vi "RT Main.vi"   [LabVIEW 2018]
doc: "Main real-time VI running on cRIO"
uses:
  Support/Message Queue/Message.ctl
  Controls/Control Mode.ctl
  Controls/Parameters.ctl
  Controls/Config.ctl
  Controls/Settings.ctl
  Controls/Timeouts.ctl
  Controls/ConfigCalibration.ctl
  Controls/ValveState.ctl
  Controls/Valve List.ctl
  Controls/ValveUpdate.ctl
  Controls/IT State.ctl
  Controls/OT State.ctl
  Controls/DL State.ctl
  Controls/BR State.ctl
  Controls/TWT State.ctl
  Controls/DLT State.ctl
  Controls/Clean State.ctl
  Controls/Actions.ctl
  Globals/Global - Configuration Options.vi
  Globals/Global - RT Stream Connections.vi
  support/Message Queue/Message Queue.lvlib
  <vilib>/nisyscfg/nisyscfg.lvlib
types:
  T1 = typedef "Message Queue.lvlib/Message.ctl" = enum16{"Initialize", "Initialize UI Refs", "Disable Controls", "Enable UI Controls", "Connect RT", "Get Control Mode from RT", "Send Control Mode to UI", "Update Control Mode", "Get Config from RT", "Send Config to UI", "Update Parameters", "Change Parameters", "Calibrate Config", "Update Calibration", "Change Valve State", "Get Valve Status from RT", "Send Valve Status to UI", "Update Valve Status", "Inital UI Values", "Disconnect RT", "Close Connection", "Disconnect UI", "Run Mode", "Stop ALL", "Change Control Mode", "Skid Manual", "Computer Manual", "Step Automated", "Fully Automated", "Reset", "Critical Error", "Log-Only Error", "Non-Critical Error", "RT Error", "Update System Status", "Update DI Status", "Clear System Status", "Update Warning", "Clear Warning", "Upate Timeout", "Update Reset Status", "Waiting", "Verify Password", "Manual Cleaning Process", "Update Manual Cleaning Process", "Exit", "---Copy This Frame---"}
  T2 = typedef "Control Mode.ctl" = enum16{"Skid Manual", "Computer Manual", "Step Automated", "Fully Automated"}
  T3 = typedef "Parameters.ctl" = cluster{"PDP (IN)":T4, "SETTINGS":T5, "TIMEOUTS (SEC)":T6}
  T4 = typedef "Config.ctl" = cluster{"TWTT OP":dbl, "TWTT PDP":dbl, "DLT OP":dbl, "DLT PDP 01":dbl, "DLT PDP 02":dbl, "BR OP":dbl, "BR TWT ALIGN":dbl, "BR DL ALIGN":dbl}
  T5 = typedef "Settings.ctl" = cluster{"HPL Low (PSI)":dbl, "HPL High (PSI)":dbl, "HPH Low (PSI)":dbl, "HPH High (PSI)":dbl, "AP Low (PSI)":dbl, "AP High (PSI)":dbl, "DL Clean (SEC)":dbl, "Reset (MIN)":dbl}
  T6 = typedef "Timeouts.ctl" = cluster{"TWTT Drive":dbl, "DL Drive":dbl, "DL Rotate":dbl, "BR Drive":dbl, "OT Engage":dbl, "PLUG Drive":dbl, "IT Engage":dbl, "IT 1REV":dbl, "IT nREV":dbl}
  T7 = typedef "ConfigCalibration.ctl" = enum16{"CAL STOP", "TWTT OP (IN)", "TWTT PDP (IN)", "DLT OP (IN)", "DLT PDP 01 (IN)", "DLT PDP 02 (IN)", "BR OP (IN)", "BR TWT ALIGN (IN)", "BR DL ALIGN (IN)"}
  T8 = typedef "ValveState.ctl" = cluster{"Valve List":T9, "State":bool}
  T9 = typedef "Valve List.ctl" = enum16{"SV-1 IT CW", "SV-1 IT CCW", "SV-2 OT CW", "SV-2 OT CCW", "SV-3 DL CW", "SV-3 DL CCW", "SV-4 BR RIGHT", "SV-4 BR LEFT", "SV-5 TWT FWD", "SV-6 TWT BWD", "SV-7 DL FWD", "SV-8 DL BWD", "SV-12 H2O PILOT", "SV-13 CLEAN AIR", "SV-15 CLEAN H2O"}
  T10 = typedef "IT State.ctl" = enum16{"IT STOP", "IT ROTATE CCW ENG", "IT ROTATE CCW QF1R", "IT CCW ENG & QF1R", "IT ROTATE CCW 2.5 REV", "IT ROTATE CW 2.5 REV", "IT CW TIGHTEN VALVE", "IT CCW PULSE", "SV-1 IT CW TRUE", "SV-1 IT CW FALSE", "SV-1 IT CCW TRUE", "SV-1 IT CCW FALSE"}
  T11 = typedef "ValveUpdate.ctl" = cluster{"Index":i32, "Valve Array":bool[]}
  T12 = typedef "OT State.ctl" = enum16{"OT STOP", "OT ROTATE CW ENG", "OT ROTATE CCW 2.5 REV", "OT ROTATE CW 2.5 REV", "OT CW TIGHTEN PLUG", "SV-2 OT CW TRUE", "SV-2 OT CW FALSE", "SV-2 OT CCW TRUE", "SV-2 OT CCW FALSE"}
  T13 = typedef "DL State.ctl" = enum16{"DL STOP", "DL ROTATE CW", "DL ROTATE CCW", "SV-3 DL CW TRUE", "SV-3 DL CW FALSE", "SV-3 DL CCW TRUE", "SV-3 DL CCW FALSE"}
  T14 = typedef "BR State.ctl" = enum16{"BR STOP", "BR DRIVE LEFT PDP", "BR LEFT ALIGN TWT", "BR DRIVE RIGHT PDP", "BR RIGHT TO INIT", "BR RIGHT FOR DL", "SV-4 BR RIGHT TRUE", "SV-4 BR RIGHT FALSE", "SV-4 BR LEFT TRUE", "SV-4 BR LEFT FALSE", "BR RESET"}
  T15 = typedef "TWT State.ctl" = enum16{"TWTT STOP", "TWTT DRIVE FWD PDP", "TWTT DRIVE BWD PDP", "TWTT BWD 0.256 IN", "TWTT FWD 0.256 IN", "TWT FWD BEFORE SCREW", "SV-5 TWTT FWD TRUE", "SV-5 TWTT FWD FALSE", "SV-6 TWTT BWD TRUE", "SV-6 TWTT BWD FALSE", "TWTT RESET"}
  T16 = typedef "DLT State.ctl" = enum16{"DLT STOP", "DLT DRIVE FWD PDP", "DLT DRIVE FWD", "DLT DRIVE BWD", "DLT DRIVE BWD PDP CLEAN", "DLT DRIVE BWD PDP", "DLT HOLD BACK", "SV-7 DLT FWD TRUE", "SV-7 DLT FWD FALSE", "SV-8 DLT BWD TRUE", "SV-8 DLT BWD FALSE", "DLT RESET"}
  T17 = typedef "Clean State.ctl" = enum16{"CLEAN STOP", "CLEAN CAMERA", "CLEAN THREADS", "CLEAN THREADS MANUAL", "SV-12 H2O PILOT TRUE", "SV-12 H2O PILOT FALSE", "SV-13 CLEAN AIR TRUE", "SV-13 CLEAN AIR FALSE", "SV-15 CLEAN H2O TRUE", "SV-15 CLEAN H2O FALSE"}
  T18 = typedef "Actions.ctl" = enum16{"Drive TWT Track FWD to PDP", "Slowly Rotate OT CW for OT ENG", "Quickly Rotate IT CCW for One REV", "Drive Bottom Rail Right to Align DL", "Drive DL Track FWD to PDP", "Screw Divert Line", "Continuous Circulation", "Unscrew Divert Line", "Drive DL Track BWD to PDP for Cleaning", "Cleaning Process", "Drive DL Track BWD to PDP", "Drive Bottom Rail Back to Align TWT", "Screw Plug Back to Sub", "Tighten Bleed Valve", "Drive TWT Track BWD to PDP", "Drive Bottom Rail Right to Init Pos", "IT ROTATE CCW 2.5 REV", "OT ROTATE CCW 2.5 REV", "OT ROTATE CW 2.5 REV", "TWTT BWD 0.265 IN", "IT ROTATE CW 2.5 REV", "TWTT FWD 0.265 IN", "OT CW TIGHTEN PLUG"}
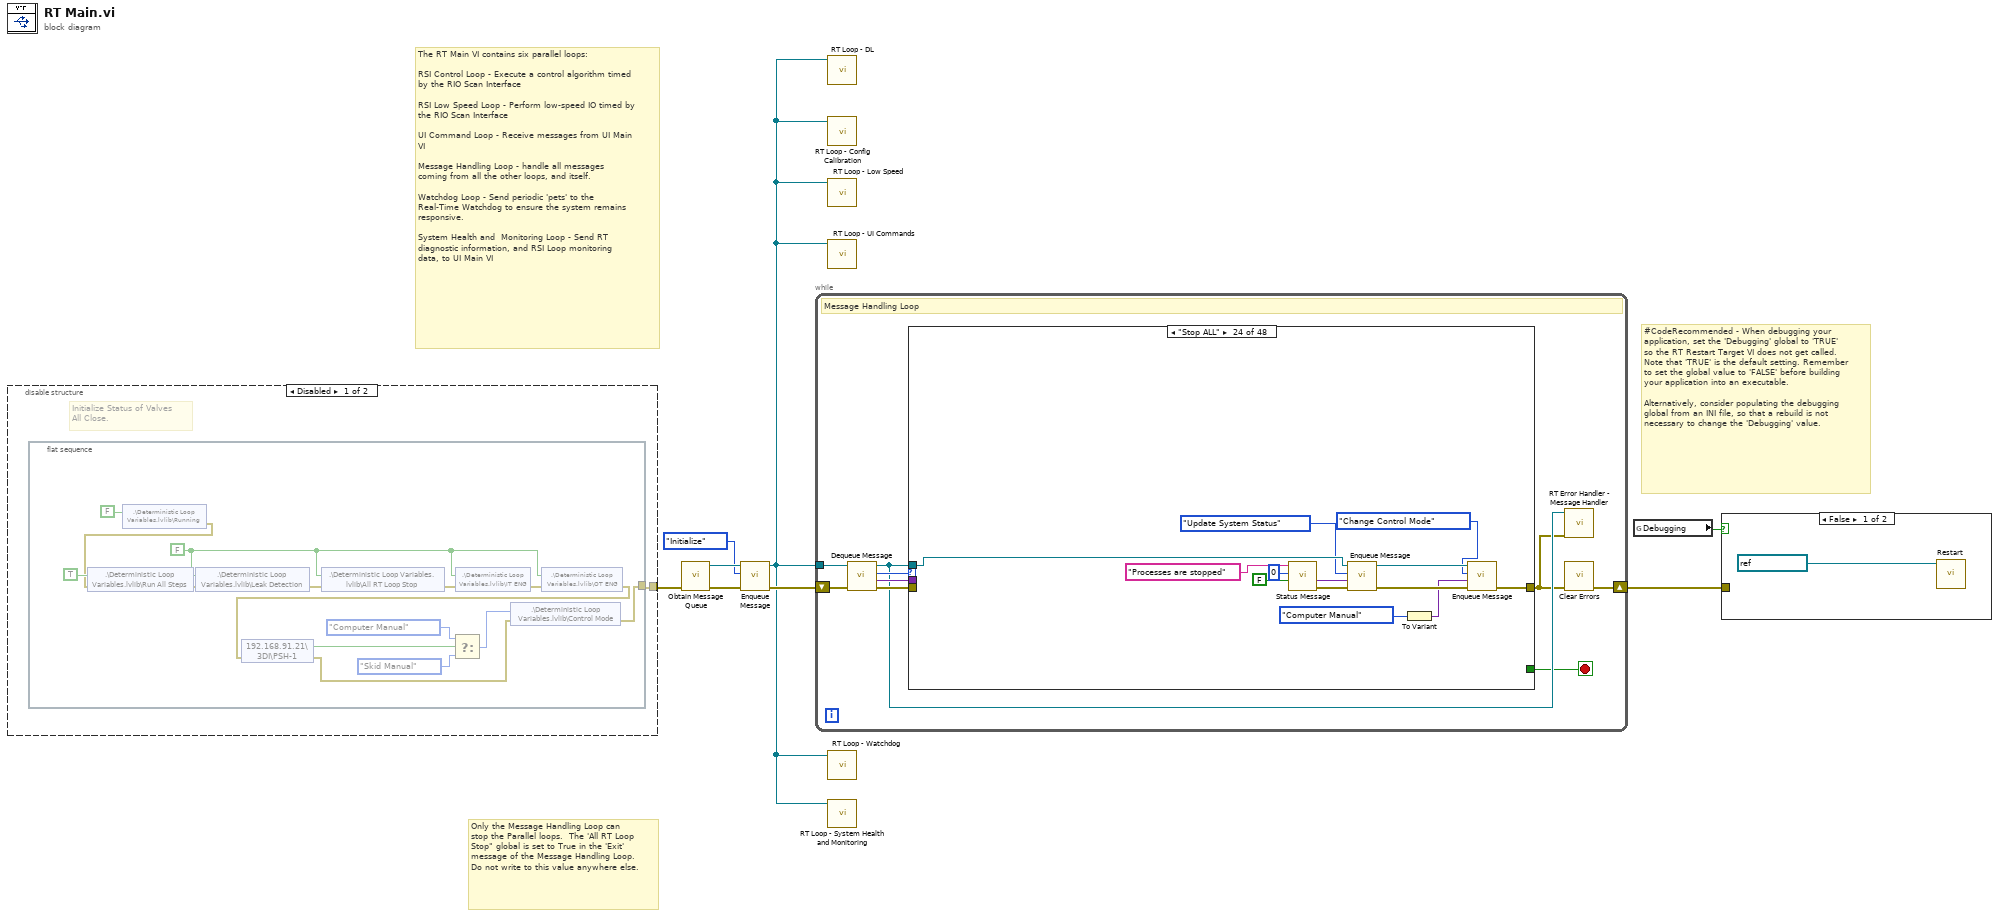
[diagram p0: block diagram]
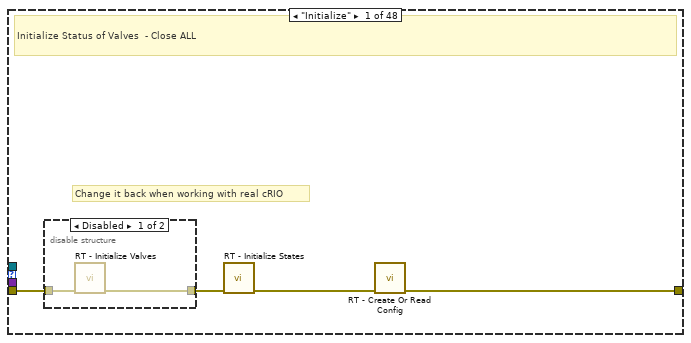
[diagram p3: hidden frame]
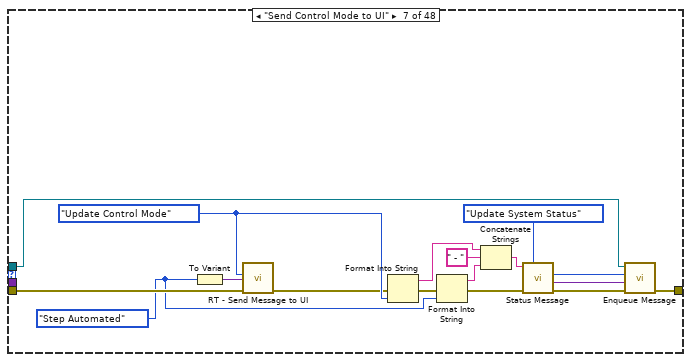
[diagram p10: hidden frame]
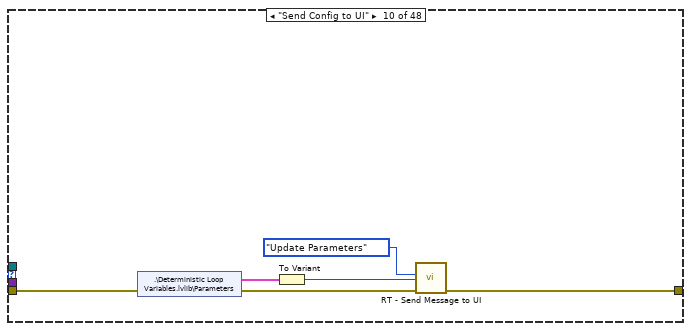
[diagram p13: hidden frame]
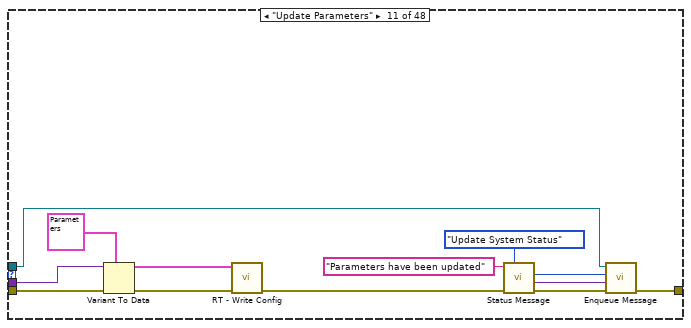
[diagram p14: hidden frame]
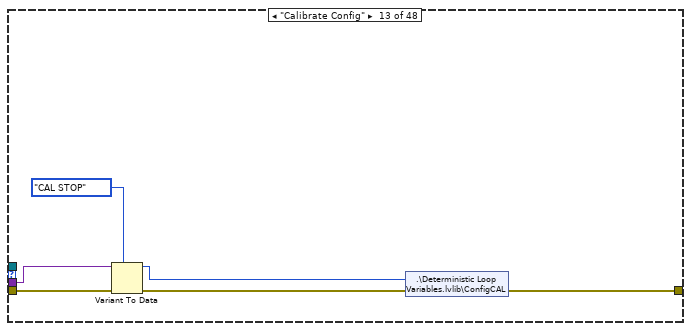
[diagram p16: hidden frame]
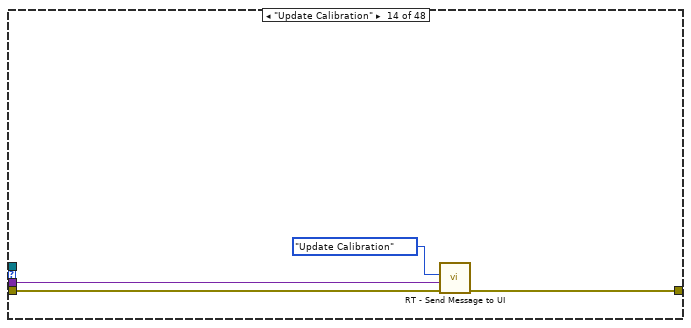
[diagram p17: hidden frame]
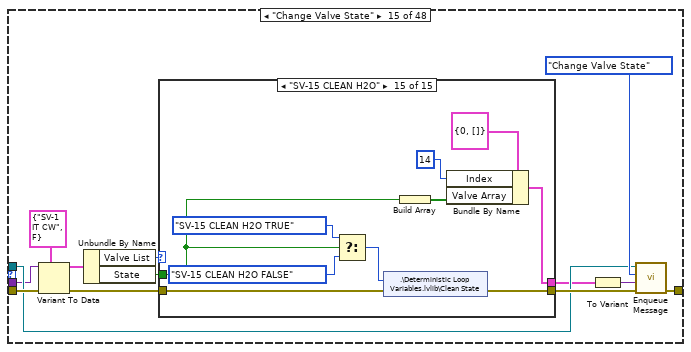
[diagram p18: hidden frame]
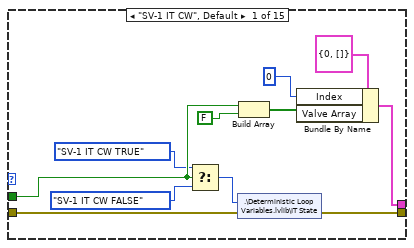
[diagram p19: hidden frame]
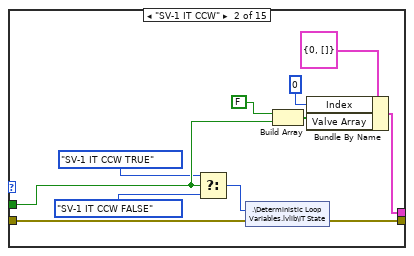
[diagram p20: hidden frame]
diagram:
  # "#CodeRecommended - When debugging your application, set the 'Debugging' global to 'TRUE' so the RT Restart Target VI does not get called.  Note that 'TRUE' is the default setting. Remember to set the global value to 'FALSE' before building your application into an executable.\n\nAlternatively, consider populating the debugging global from an INI file, so that a rebuild is not necessary to change the 'Debugging' value."
  # "Only the Message Handling Loop can stop the Parallel loops.  The 'All RT Loop Stop\" global is set to True in the 'Exit' message of the Message Handling Loop.  Do not write to this value anywhere else."
  # "The RT Main VI contains six parallel loops:\n\nRSI Control Loop - Execute a control algorithm timed by the RIO Scan Interface\n\nRSI Low Speed Loop - Perform low-speed IO timed by the RIO Scan Interface\n\nUI Command Loop - Receive messages from UI Main VI\n\nMessage Handling Loop - handle all messages coming from all the other loops, and itself.\n\nWatchdog Loop - Send periodic 'pets' to the Real-Time Watchdog to ensure the system remains responsive.\n\nSystem Health and  Monitoring Loop - Send RT diagnostic information, and RSI Loop monitoring data, to UI Main VI"
  n1 = disable-structure shown="Disabled" {
    disable-tunnel: [w9 _] -> w8
    frame Disabled {
      # "Initialize Status of Valves\nAll Close."
      n2 = flat-sequence {
        tunnel: [w18] -> w9
        frame #0 {
          w19 = FALSE ("All RT Loop Stop")
          n3 = shared-variable ".\\Deterministic Loop Variables.lvlib\\Running"(FALSE ("Running")) -> (error out=w11:errorcluster)  [unwired: 1 in]
          n4 = shared-variable ".\\Deterministic Loop Variables.lvlib\\Run All Steps"(TRUE ("Auto Mode"), error in=w11) -> (error out=w21:errorcluster)
          n5 = shared-variable ".\\Deterministic Loop Variables.lvlib\\Leak Detection"(w19, error in=w21) -> (error out=w20:errorcluster)
          n6 = shared-variable ".\\Deterministic Loop Variables.lvlib\\All RT Loop Stop"(w19, error in=w20) -> (error out=w24:errorcluster)
          n7 = shared-variable ".\\Deterministic Loop Variables.lvlib\\IT ENG"(w19, error in=w24) -> (error out=w23:errorcluster)
          n8 = shared-variable ".\\Deterministic Loop Variables.lvlib\\OT ENG"(w19, error in=w23) -> (error out=w12:errorcluster)
          n9 = shared-variable "192.168.91.21\\3DI\\PSH-1"(error in=w12) -> (w13:bool, error out=w14:errorcluster)
          n10 = Select(t=Control_Mode."Computer Manual" ("Control Mode"), s=w13, f=Control_Mode."Skid Manual") -> (s? t:f=w15:T2)
          n11 = shared-variable ".\\Deterministic Loop Variables.lvlib\\Control Mode"(w15, error in=w14) -> (error out=w18:errorcluster)
        }
      }
    }
    frame Enabled {
    }
  }
  n12 = call "Obtain Message Queue.vi"("error in (no error)"=w8) -> ("error out"=w6:errorcluster, "Message Queue"=w7:refnum<queue>)  [unwired: 9 in]
  n13 = call "Enqueue Message.vi"("error in (no error)"=w6, "Message"=Message."Initialize", "Message Queue"=w7) -> ("error out"=w4:errorcluster, "dup Message Queue"=w1:refnum<queue>)  [unwired: 7 in]
  n14 = while {
    tunnel: w1 -> [w33]
    shift-right: [w28] -> w3
    shift-left: w4 -> [w32]
    stop <- w26 stop-if-true
    # "Message Handling Loop"
    n15 = call "Dequeue Message.vi"("error in (no error)"=w32, "Message Queue"=w33) -> ("error out"=w29:errorcluster, "Message Data"=w30:variant, "Message"=w31:T1, "dup Message Queue"=w27:refnum<queue>)  [unwired: 6 in]
    n16 = case shown="\"Stop ALL\"" w31 {
      selector: w31 -> [_ _ _ _ _ _ _ _ _ _ _ _ _ _ _ _ _ _ _ _ _ _ _ _ _ _ _ _ _ _ _ _ _ _ _ _ _ _ _ _ _ _ _ _ _ _ _ w401]
      tunnel: w30 -> [_ _ _ _ _ _ _ _ _ _ w81 _ w88 w89 w95 _ _ _ _ _ _ _ w280 _ w309 _ _ _ _ _ _ _ _ _ w340 w344 _ w349 _ w354 w357 w370 _ _ w382 _ _ _]
      tunnel: w29 -> [w37 w41 w42 w43 w44 w45 w47 w62 w63 w65 w80 w82 w87 w91 w105 w268 w269 w270 w271 w272 w273 w274 w278 _ w308 w311 w312 w313 w314 w328 w335 w336 w337 w338 w342 w346 w347 w351 w352 w356 w359 w369 w376 w378 w381 w393 w396 _]
      tunnel: w27 -> [_ _ _ _ _ _ w48 _ _ _ w75 _ _ _ w96 _ _ _ _ _ _ _ _ w293 w310 _ _ _ _ w326 _ _ _ _ _ _ _ _ _ _ _ w362 _ _ _ w394 _ _]
      tunnel: [w36 w41 w42 w43 w44 w45 w59 w62 w63 w67 w77 w82 w83 w90 w98 w268 w269 w270 w271 w272 w273 w274 w275 w285 w294 w311 w312 w313 w314 w315 w335 w336 w337 w338 w341 w345 w347 w350 w352 w355 w358 w363 w376 w377 w380 w385 w396 w397] -> w25
      tunnel: [_ _ _ _ _ _ _ _ _ _ _ _ _ _ _ _ _ _ _ _ _ _ _ _ _ _ _ _ _ _ _ _ _ _ _ _ _ _ _ _ _ _ _ _ _ TRUE _ _] -> w26
      frame "Initialize" {
        # "Change it back when working with real cRIO"
        # "Initialize Status of Valves  - Close ALL"
        n17 = disable-structure shown="Disabled" {
          disable-tunnel: w37 -> [w39 w40]
          disable-tunnel: [w38 w40] -> w35
          frame Disabled {
            n18 = call "RT - Initialize Valves.vi"("error in"=w39) -> ("error out"=w38:errorcluster)  [unwired: 10 in]
          }
          frame Enabled {
          }
        }
        n19 = call "RT - Initialize States.vi"("error in"=w35) -> ("error out"=w34:errorcluster)  [unwired: 10 in]
        n20 = call "RT - Create Or Read Config.vi"("error in"=w34) -> ("error out"=w36:errorcluster)  [unwired: 10 in]
      }
      frame "Initialize UI Refs" {
      }
      frame "Disable Controls" {
      }
      frame "Enable UI Controls" {
      }
      frame "Connect RT" {
      }
      frame "Get Control Mode from RT" {
      }
      frame "Send Control Mode to UI" {
        w46 = Control_Mode."Step Automated" ("Control Mode")
        w54 = Message."Update Control Mode" ("Message")
        n21 = To Variant(anything=w46) -> (Variant=w61:variant)
        n22 = call "RT - Send Message to UI.vi"("error in (no error)"=w47, "Message Data"=w61, "Message"=w54) -> ("error out"=w51:errorcluster)  [unwired: 8 in]
        n23 = Format Into String(error in=w51, w54) -> (resulting string=w53:string, error out=w50:errorcluster)  [unwired: 2 in]
        n24 = Format Into String(error in=w50, w46) -> (resulting string=w52:string, error out=w49:errorcluster)  [unwired: 2 in]
        n25 = Concatenate Strings(w53, " - " ("string"), w52) -> (w57:string)
        n26 = call "Status Message.vi"("Error In"=w49, "Message"=w57) -> ("Error Out"=w56:errorcluster, "Status"=w55:variant)  [unwired: 7 in]
        n27 = call "Enqueue Message.vi"("error in (no error)"=w56, "Message Data"=w55, "Message"=Message."Update System Status", "Message Queue"=w48) -> ("error out"=w59:errorcluster)  [unwired: 6 in, 1 out]
      }
      frame "Update Control Mode" {
        # "Update Control Configurations - Send the specified Control Configuration values to the RSI Control Loop"
      }
      frame "Get Config from RT" {
      }
      frame "Send Config to UI" {
        n28 = shared-variable ".\\Deterministic Loop Variables.lvlib\\Parameters"(error in=w65) -> (w66:T3, error out=w64:errorcluster)
        n29 = To Variant(anything=w66) -> (Variant=w68:variant)
        n30 = call "RT - Send Message to UI.vi"("error in (no error)"=w64, "Message Data"=w68, "Message"=Message."Update Parameters") -> ("error out"=w67:errorcluster)  [unwired: 8 in]
      }
      frame "Update Parameters" {
        n31 = Variant To Data(error in=w80, type=T3 {"PDP (IN)"={"TWTT OP"=0.0, "TWTT PDP"=0.0, "DLT OP"=0.0, "DLT PDP 01"=0.0, "DLT PDP 02"=0.0, "BR OP"=0.0, "BR TWT ALIGN"=0.0, "BR DL ALIGN"=0.0}, "SETTINGS"={"HPL Low (PSI)"=0.0, "HPL High (PSI)"=0.0, "HPH Low (PSI)"=0.0, "HPH High (PSI)"=0.0, "AP Low (PSI)"=0.0, "AP High (PSI)"=0.0, "DL Clean (SEC)"=4.0, "Reset (MIN)"=2.0}, "TIMEOUTS (SEC)"={"TWTT Drive"=20.0, "DL Drive"=20.0, "DL Rotate"=60.0, "BR Drive"=20.0, "OT Engage"=20.0, "PLUG Drive"=60.0, "IT Engage"=20.0, "IT 1REV"=30.0, "IT nREV"=60.0}} ("PARAMETERS"), Variant=w81) -> (data=w71:T3, error out=w73:errorcluster)
        n32 = call "RT - Write Config.vi"("error in"=w73, "PARAMETERS"=w71) -> ("error out"=w72:errorcluster)  [unwired: 9 in]
        n33 = call "Status Message.vi"("Error In"=w72, "Message"="Parameters have been updated") -> ("Error Out"=w76:errorcluster, "Status"=w78:variant)  [unwired: 7 in]
        n34 = call "Enqueue Message.vi"("error in (no error)"=w76, "Message Data"=w78, "Message"=Message."Update System Status", "Message Queue"=w75) -> ("error out"=w77:errorcluster)  [unwired: 6 in, 1 out]
      }
      frame "Change Parameters" {
      }
      frame "Calibrate Config" {
        n35 = Variant To Data(error in=w87, type=ConfigCalibration."CAL STOP" ("ConfigCAL"), Variant=w88) -> (data=w85:T7, error out=w84:errorcluster)
        n36 = shared-variable ".\\Deterministic Loop Variables.lvlib\\ConfigCAL"(w85, error in=w84) -> (error out=w83:errorcluster)
      }
      frame "Update Calibration" {
        n37 = call "RT - Send Message to UI.vi"("error in (no error)"=w91, "Message Data"=w89, "Message"=Message."Update Calibration") -> ("error out"=w90:errorcluster)  [unwired: 8 in]
      }
      frame "Change Valve State" {
        n38 = Variant To Data(error in=w105, type=T8 {"Valve List"=enum."SV-1 IT CW", "State"=FALSE} ("TWT State"), Variant=w95) -> (data=w102:T8, error out=w103:errorcluster)
        n39 = Unbundle By Name(w102) -> ("Valve List"=w101:T9, "State"=w100:bool)
        n40 = case shown="\"SV-15 CLEAN H2O\"" w101 {
          tunnel: w103 -> [w115 w126 w137 w148 w159 w170 w181 w192 w203 w214 w225 w236 w246 w256 w266]
          tunnel: [w116 w127 w138 w149 w160 w171 w182 w193 w204 w215 w226 w237 w247 w257 w267] -> w99
          tunnel: w100 -> [w110 w122 w134 w144 w154 w163 w176 w186 w198 w209 w220 w231 w241 w251 w261]
          tunnel: [w109 w121 w135 w142 w156 w167 w178 w189 w200 w211 w222 w233 w243 w253 w263] -> w93
          frame "SV-1 IT CW", Default {
            n41 = Select(t=IT_State."SV-1 IT CW TRUE" ("IT State"), s=w110, f=IT_State."SV-1 IT CW FALSE" ("IT State")) -> (s? t:f=w114:T10)
            n42 = shared-variable ".\\Deterministic Loop Variables.lvlib\\IT State"(w114, error in=w115) -> (error out=w116:errorcluster)
            n43 = Build Array(w110, FALSE ("element")) -> (w111:bool[])
            n44 = Bundle By Name(cluster=T11 {"Index"=0, "Valve Array"=[]} ("ValveUpdate"), "Index"=0, "Valve Array"=w111) -> (w109:T11)
          }
          frame "SV-1 IT CCW" {
            n45 = Select(t=IT_State."SV-1 IT CCW TRUE" ("IT State"), s=w122, f=IT_State."SV-1 IT CCW FALSE" ("IT State")) -> (s? t:f=w117:T10)
            n46 = shared-variable ".\\Deterministic Loop Variables.lvlib\\IT State"(w117, error in=w126) -> (error out=w127:errorcluster)
            n47 = Build Array(FALSE ("element"), w122) -> (w124:bool[])
            n48 = Bundle By Name(cluster=T11 {"Index"=0, "Valve Array"=[]} ("ValveUpdate"), "Index"=0, "Valve Array"=w124) -> (w121:T11)
          }
          frame "SV-2 OT CW" {
            n49 = Select(t=OT_State."SV-2 OT CW TRUE" ("OT State"), s=w134, f=OT_State."SV-2 OT CW FALSE" ("OT State")) -> (s? t:f=w128:T12)
            n50 = Build Array(w134, FALSE ("element")) -> (w132:bool[])
            n51 = shared-variable ".\\Deterministic Loop Variables.lvlib\\OT State"(w128, error in=w137) -> (error out=w138:errorcluster)
            n52 = Bundle By Name(cluster=T11 {"Index"=0, "Valve Array"=[]} ("ValveUpdate"), "Index"=2, "Valve Array"=w132) -> (w135:T11)
          }
          frame "SV-2 OT CCW" {
            n53 = Select(t=OT_State."SV-2 OT CCW TRUE" ("OT State"), s=w144, f=OT_State."SV-2 OT CCW FALSE" ("OT State")) -> (s? t:f=w147:T12)
            n54 = shared-variable ".\\Deterministic Loop Variables.lvlib\\OT State"(w147, error in=w148) -> (error out=w149:errorcluster)
            n55 = Build Array(FALSE ("element"), w144) -> (w145:bool[])
            n56 = Bundle By Name(cluster=T11 {"Index"=0, "Valve Array"=[]} ("ValveUpdate"), "Index"=2, "Valve Array"=w145) -> (w142:T11)
          }
          frame "SV-3 DL CW" {
            n57 = Select(t=DL_State."SV-3 DL CW TRUE" ("DL State"), s=w154, f=DL_State."SV-3 DL CW FALSE" ("DL State")) -> (s? t:f=w150:T13)
            n58 = shared-variable ".\\Deterministic Loop Variables.lvlib\\DL State"(w150, error in=w159) -> (error out=w160:errorcluster)
            n59 = Build Array(w154, FALSE ("element")) -> (w157:bool[])
            n60 = Bundle By Name(cluster=T11 {"Index"=0, "Valve Array"=[]} ("ValveUpdate"), "Index"=4, "Valve Array"=w157) -> (w156:T11)
          }
          frame "SV-3 DL CCW" {
            n61 = Select(t=DL_State."SV-3 DL CCW TRUE" ("DL State"), s=w163, f=DL_State."SV-3 DL CCW FALSE" ("DL State")) -> (s? t:f=w165:T13)
            n62 = shared-variable ".\\Deterministic Loop Variables.lvlib\\DL State"(w165, error in=w170) -> (error out=w171:errorcluster)
            n63 = Build Array(FALSE ("element"), w163) -> (w168:bool[])
            n64 = Bundle By Name(cluster=T11 {"Index"=0, "Valve Array"=[]} ("ValveUpdate"), "Index"=4, "Valve Array"=w168) -> (w167:T11)
          }
          frame "SV-4 BR RIGHT" {
            n65 = Select(t=BR_State."SV-4 BR RIGHT TRUE" ("BR State"), s=w176, f=BR_State."SV-4 BR RIGHT FALSE" ("BR State")) -> (s? t:f=w172:T14)
            n66 = Build Array(w176, FALSE ("element")) -> (w179:bool[])
            n67 = shared-variable ".\\Deterministic Loop Variables.lvlib\\BR State"(w172, error in=w181) -> (error out=w182:errorcluster)
            n68 = Bundle By Name(cluster=T11 {"Index"=0, "Valve Array"=[]} ("ValveUpdate"), "Index"=6, "Valve Array"=w179) -> (w178:T11)
          }
          frame "SV-4 BR LEFT" {
            n69 = Select(t=BR_State."SV-4 BR LEFT TRUE" ("BR State"), s=w186, f=BR_State."SV-4 BR LEFT FALSE" ("BR State")) -> (s? t:f=w183:T14)
            n70 = shared-variable ".\\Deterministic Loop Variables.lvlib\\BR State"(w183, error in=w192) -> (error out=w193:errorcluster)
            n71 = Build Array(FALSE ("element"), w186) -> (w190:bool[])
            n72 = Bundle By Name(cluster=T11 {"Index"=0, "Valve Array"=[]} ("ValveUpdate"), "Index"=6, "Valve Array"=w190) -> (w189:T11)
          }
          frame "SV-5 TWT FWD" {
            n73 = Select(t=TWT_State."SV-5 TWTT FWD TRUE" ("TWTT State"), s=w198, f=TWT_State."SV-5 TWTT FWD FALSE" ("TWTT State")) -> (s? t:f=w194:T15)
            n74 = shared-variable ".\\Deterministic Loop Variables.lvlib\\TWTT State"(w194, error in=w203) -> (error out=w204:errorcluster)
            n75 = Build Array(w198, FALSE ("element")) -> (w201:bool[])
            n76 = Bundle By Name(cluster=T11 {"Index"=0, "Valve Array"=[]} ("ValveUpdate"), "Index"=8, "Valve Array"=w201) -> (w200:T11)
          }
          frame "SV-6 TWT BWD" {
            n77 = Select(t=TWT_State."SV-6 TWTT BWD TRUE" ("TWTT State"), s=w209, f=TWT_State."SV-6 TWTT BWD FALSE" ("TWTT State")) -> (s? t:f=w208:T15)
            n78 = shared-variable ".\\Deterministic Loop Variables.lvlib\\TWTT State"(w208, error in=w214) -> (error out=w215:errorcluster)
            n79 = Build Array(FALSE ("element"), w209) -> (w212:bool[])
            n80 = Bundle By Name(cluster=T11 {"Index"=0, "Valve Array"=[]} ("ValveUpdate"), "Index"=8, "Valve Array"=w212) -> (w211:T11)
          }
          frame "SV-7 DL FWD" {
            n81 = Select(t=DLT_State."SV-7 DLT FWD TRUE" ("DLT State"), s=w220, f=DLT_State."SV-7 DLT FWD FALSE" ("DLT State")) -> (s? t:f=w216:T16)
            n82 = shared-variable ".\\Deterministic Loop Variables.lvlib\\DLT State"(w216, error in=w225) -> (error out=w226:errorcluster)
            n83 = Build Array(w220, FALSE ("element")) -> (w223:bool[])
            n84 = Bundle By Name(cluster=T11 {"Index"=0, "Valve Array"=[]} ("ValveUpdate"), "Index"=10, "Valve Array"=w223) -> (w222:T11)
          }
          frame "SV-8 DL BWD" {
            n85 = Select(t=DLT_State."SV-8 DLT BWD TRUE" ("DLT State"), s=w231, f=DLT_State."SV-8 DLT BWD FALSE" ("DLT State")) -> (s? t:f=w227:T16)
            n86 = shared-variable ".\\Deterministic Loop Variables.lvlib\\DLT State"(w227, error in=w236) -> (error out=w237:errorcluster)
            n87 = Build Array(FALSE ("element"), w231) -> (w234:bool[])
            n88 = Bundle By Name(cluster=T11 {"Index"=0, "Valve Array"=[]} ("ValveUpdate"), "Index"=10, "Valve Array"=w234) -> (w233:T11)
          }
          frame "SV-12 H2O PILOT" {
            n89 = Select(t=Clean_State."SV-12 H2O PILOT TRUE" ("Clean State"), s=w241, f=Clean_State."SV-12 H2O PILOT FALSE" ("Clean State")) -> (s? t:f=w238:T17)
            n90 = shared-variable ".\\Deterministic Loop Variables.lvlib\\Clean State"(w238, error in=w246) -> (error out=w247:errorcluster)
            n91 = Build Array(w241) -> (w244:bool[])
            n92 = Bundle By Name(cluster=T11 {"Index"=0, "Valve Array"=[]} ("ValveUpdate"), "Index"=12, "Valve Array"=w244) -> (w243:T11)
          }
          frame "SV-13 CLEAN AIR" {
            n93 = Select(t=Clean_State."SV-13 CLEAN AIR TRUE" ("Clean State"), s=w251, f=Clean_State."SV-13 CLEAN AIR FALSE" ("Clean State")) -> (s? t:f=w248:T17)
            n94 = shared-variable ".\\Deterministic Loop Variables.lvlib\\Clean State"(w248, error in=w256) -> (error out=w257:errorcluster)
            n95 = Build Array(w251) -> (w254:bool[])
            n96 = Bundle By Name(cluster=T11 {"Index"=0, "Valve Array"=[]} ("ValveUpdate"), "Index"=13, "Valve Array"=w254) -> (w253:T11)
          }
          frame "SV-15 CLEAN H2O" {
            n97 = Select(t=Clean_State."SV-15 CLEAN H2O TRUE" ("Clean State"), s=w261, f=Clean_State."SV-15 CLEAN H2O FALSE" ("Clean State")) -> (s? t:f=w258:T17)
            n98 = shared-variable ".\\Deterministic Loop Variables.lvlib\\Clean State"(w258, error in=w266) -> (error out=w267:errorcluster)
            n99 = Build Array(w261) -> (w264:bool[])
            n100 = Bundle By Name(cluster=T11 {"Index"=0, "Valve Array"=[]} ("ValveUpdate"), "Index"=14, "Valve Array"=w264) -> (w263:T11)
          }
        }
        n101 = To Variant(anything=w93) -> (Variant=w94:variant)
        n102 = call "Enqueue Message.vi"("error in (no error)"=w99, "Message Data"=w94, "Message"=Message."Change Valve State", "Message Queue"=w96) -> ("error out"=w98:errorcluster)  [unwired: 6 in, 1 out]
      }
      frame "Get Valve Status from RT" {
      }
      frame "Send Valve Status to UI" {
      }
      frame "Update Valve Status" {
      }
      frame "Inital UI Values" {
      }
      frame "Disconnect RT" {
      }
      frame "Close Connection" {
      }
      frame "Disconnect UI" {
      }
      frame "Run Mode" {
        n103 = Variant To Data(error in=w278, type=TRUE, Variant=w280) -> (data=w277:bool, error out=w276:errorcluster)
        n104 = shared-variable ".\\Deterministic Loop Variables.lvlib\\Running"(w277, error in=w276) -> (error out=w275:errorcluster)
      }
      frame "Stop ALL" {
        n105 = call "Status Message.vi"("Start/End"=FALSE, "Step #"=0, "Message"="Processes are stopped") -> ("Error Out"=w290:errorcluster, "Status"=w291:variant)  [unwired: 6 in]
        n106 = call "Enqueue Message.vi"("error in (no error)"=w290, "Message Data"=w291, "Message"=Message."Update System Status", "Message Queue"=w293) -> ("error out"=w286:errorcluster, "dup Message Queue"=w284:refnum<queue>)  [unwired: 6 in]
        n107 = To Variant(anything=Control_Mode."Computer Manual" ("Control Mode")) -> (Variant=w281:variant)
        n108 = call "Enqueue Message.vi"("error in (no error)"=w286, "Message Data"=w281, "Message"=Message."Change Control Mode", "Message Queue"=w284) -> ("error out"=w285:errorcluster)  [unwired: 6 in, 1 out]
      }
      frame "Change Control Mode" {
        w297 = FALSE ("All RT Loop Stop")
        n109 = Variant To Data(error in=w308, type=Control_Mode."Skid Manual" ("Control Mode"), Variant=w309) -> (data=w304:T2, error out=w303:errorcluster)
        n110 = shared-variable ".\\Deterministic Loop Variables.lvlib\\Control Mode"(w304, error in=w303) -> (error out=w302:errorcluster)
        n111 = Equal?(x=Control_Mode."Fully Automated" ("Control Mode"), y=w304) -> (x = y?=w307:bool)
        n112 = call "Enqueue Message.vi"("error in (no error)"=w302, "Message"=Message."Send Control Mode to UI", "Message Queue"=w310) -> ("error out"=w296:errorcluster)  [unwired: 7 in, 1 out]
        n113 = shared-variable ".\\Deterministic Loop Variables.lvlib\\Run All Steps"(w307, error in=w296) -> (error out=w300:errorcluster)
        n114 = shared-variable ".\\Deterministic Loop Variables.lvlib\\Leak Detection"(w297, error in=w300) -> (error out=w299:errorcluster)
        n115 = shared-variable ".\\Deterministic Loop Variables.lvlib\\IT ENG"(w297, error in=w299) -> (error out=w298:errorcluster)
        n116 = shared-variable ".\\Deterministic Loop Variables.lvlib\\OT ENG"(w297, error in=w298) -> (error out=w295:errorcluster)
        n117 = call "RT - Initialize States.vi"("error in"=w295) -> ("error out"=w294:errorcluster)  [unwired: 10 in]
      }
      frame "Skid Manual" {
      }
      frame "Computer Manual" {
      }
      frame "Step Automated" {
      }
      frame "Fully Automated" {
      }
      frame "Reset" {
        n118 = call "Status Message.vi"("Error In"=w328, "Start/End"=FALSE, "Step #"=0, "Message"="Machine Control Mode Reset - START") -> ("Error Out"=w332:errorcluster, "Status"=w333:variant)  [unwired: 5 in]
        n119 = call "Enqueue Message.vi"("error in (no error)"=w332, "Message Data"=w333, "Message"=Message."Update System Status", "Message Queue"=w326) -> ("error out"=w327:errorcluster, "dup Message Queue"=w325:refnum<queue>)  [unwired: 6 in]
        n120 = To Variant(anything=TRUE) -> (Variant=w322:variant)
        n121 = call "Enqueue Message.vi"("error in (no error)"=w327, "Message Data"=w322, "Message"=Message."Update Reset Status", "Message Queue"=w325) -> ("error out"=w320:errorcluster)  [unwired: 6 in, 1 out]
        n122 = shared-variable ".\\Deterministic Loop Variables.lvlib\\Running"(FALSE ("Running"), error in=w320) -> (error out=w318:errorcluster)
        n123 = shared-variable ".\\Deterministic Loop Variables.lvlib\\Run All Steps"(TRUE ("Auto Mode"), error in=w318) -> (error out=w316:errorcluster)
        n124 = shared-variable ".\\Deterministic Loop Variables.lvlib\\Control Mode"(Control_Mode."Fully Automated" ("Control Mode"), error in=w316) -> (error out=w315:errorcluster)
      }
      frame "Critical Error" {
      }
      frame "Log-Only Error" {
      }
      frame "Non-Critical Error" {
      }
      frame "RT Error" {
      }
      frame "Update System Status" {
        n125 = call "RT - Send Message to UI.vi"("error in (no error)"=w342, "Message Data"=w340, "Message"=Message."Update System Status") -> ("error out"=w341:errorcluster)  [unwired: 8 in]
      }
      frame "Update DI Status" {
        n126 = call "RT - Send Message to UI.vi"("error in (no error)"=w346, "Message Data"=w344, "Message"=Message."Update DI Status") -> ("error out"=w345:errorcluster)  [unwired: 8 in]
      }
      frame "Clear System Status" {
      }
      frame "Update Warning" {
        n127 = call "RT - Send Message to UI.vi"("error in (no error)"=w351, "Message Data"=w349, "Message"=Message."Update Warning") -> ("error out"=w350:errorcluster)  [unwired: 8 in]
      }
      frame "Clear Warning" {
      }
      frame "Upate Timeout" {
        n128 = call "RT - Send Message to UI.vi"("error in (no error)"=w356, "Message Data"=w354, "Message"=Message."Upate Timeout") -> ("error out"=w355:errorcluster)  [unwired: 8 in]
      }
      frame "Update Reset Status" {
        n129 = call "RT - Send Message to UI.vi"("error in (no error)"=w359, "Message Data"=w357, "Message"=Message."Update Reset Status") -> ("error out"=w358:errorcluster)  [unwired: 8 in]
      }
      frame "Waiting" {
        n130 = Variant To Data(error in=w369, type=Actions."IT ROTATE CCW 2.5 REV" ("ACTIONS"), Variant=w370) -> (data=w364:T18, error out=w367:errorcluster)
        n131 = flat-sequence {
          tunnel: w367 -> [w374]
          tunnel: [w374] -> w366
          tunnel: [w373] -> w365
          tunnel: w364 -> [w373]
          tunnel: w362 -> [w371]
          tunnel: [w371] -> w361
          tunnel: w366 -> [w375]
          tunnel: w365 -> [_]
          tunnel: [w375] -> w363
          tunnel: w361 -> [_]
          frame #0 {
            n132 = Wait (ms)(milliseconds to wait=u32 1000) -> ()  [unwired: 1 out]
          }
          frame #1 {
          }
        }
      }
      frame "Verify Password" {
      }
      frame "Manual Cleaning Process" {
        n133 = shared-variable ".\\Deterministic Loop Variables.lvlib\\Clean State"(Clean_State."CLEAN THREADS MANUAL" ("Clean State"), error in=w378) -> (error out=w377:errorcluster)
      }
      frame "Update Manual Cleaning Process" {
        n134 = call "RT - Send Message to UI.vi"("error in (no error)"=w381, "Message Data"=w382, "Message"=Message."Update Manual Cleaning Process") -> ("error out"=w380:errorcluster)  [unwired: 8 in]
      }
      frame "Exit" {
        # "Destroy streams on exit"
        # "Flush the Writer Stream to ensure all pending messages are sent to UI Main VI"
        # "Stop All Parallel Loops"
        # "Release the message queue reference"
        # "Stop Message Handling Loop"
        n135 = global read "Global - RT Stream Connections.vi" "UI Writer Stream"() -> (w388:refnum<k21>)
        n136 = global read "Global - RT Stream Connections.vi" "RT Writer Stream"() -> (w391:refnum<k21>)
        n137 = Release Queue(queue=w394, error in (no error)=w393) -> (error out=w386:errorcluster)  [unwired: 1 in, 2 out]
        n138 = Flush Stream(11:w391) -> (0:w390:errorcluster, 3:w389:refnum<k21>)  [unwired: 3 in, 1 out]
        n139 = Destroy Stream Endpoint(8:w390, 11:w389) -> (0:w387:errorcluster)
        n140 = Destroy Stream Endpoint(8:w387, 11:w388) -> (0:w384:errorcluster)
        n141 = Merge Errors(w384, w386) -> (w385:errorcluster)
        n142 = shared-variable ".\\Deterministic Loop Variables.lvlib\\All RT Loop Stop"(TRUE ("All RT Loop Stop")) -> ()  [unwired: 1 in, 1 out]
      }
      frame "---Copy This Frame---" {
      }
      frame Default {
        # "'Default' case only runs if there is a message that isn't defined in any of the other cases.  Output a programming error."
        n143 = Format Into String(format string="The invalid message string \"%s\" was received in the Message Handling Loop." ("Unknown Message Error Text"), w401) -> (resulting string=w399:string)  [unwired: 2 in, 1 out]
        n144 = call <vilib>:"Error Cluster From Error Code.vi"("error message (\"\")"=w399, "error code (0)"=1) -> ("error out"=w397:errorcluster)  [unwired: 7 in]
      }
    }
    n145 = call "RT Error Handler - Message Handler.vi"("error in (no error)"=w25, "Message Queue"=w27) -> ()  [unwired: 9 in, 1 out]
    n146 = call <vilib>:"Clear Errors.vi"("error in (no error)"=w25) -> ("error out"=w28:errorcluster)  [unwired: 5 in, 1 out]
  }
  n147 = call "RT Loop - DL.vi"("Message Queue"=w1) -> ()  [unwired: 11 in]
  n148 = call "RT Loop - Config Calibration.vi"("Message Queue"=w1) -> ()  [unwired: 11 in]
  n149 = call "RT Loop - Low Speed.vi"("Message Queue"=w1) -> ()  [unwired: 11 in]
  n150 = call "RT Loop - UI Commands.vi"("Message Queue"=w1) -> ()  [unwired: 11 in]
  n151 = call "RT Loop - Watchdog.vi"("Message Queue"=w1) -> ()  [unwired: 11 in]
  n152 = call "RT Loop - System Health and Monitoring.vi"("Message Queue"=w1) -> ()  [unwired: 11 in]
  n153 = global read "Global - Configuration Options.vi" "Debugging"() -> (w2:bool)
  n154 = case shown="False" w2 {
    tunnel: w3 -> [_ _]
    frame False {
      n155 = call <vilib>:"Restart.vi"("Session in"=refnum<k21> "localhost" ("session in")) -> ()  [unwired: 8 in, 3 out]
    }
    frame True {
    }
  }
